vi "Boolean Debounce.vi"(1 "Reset":bool, 2 "Miliseconds":dbl, 3 "In":bool) -> (0 "Debounced":bool)   [LabVIEW 2016]
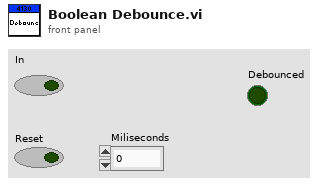
[diagram p1: front panel]
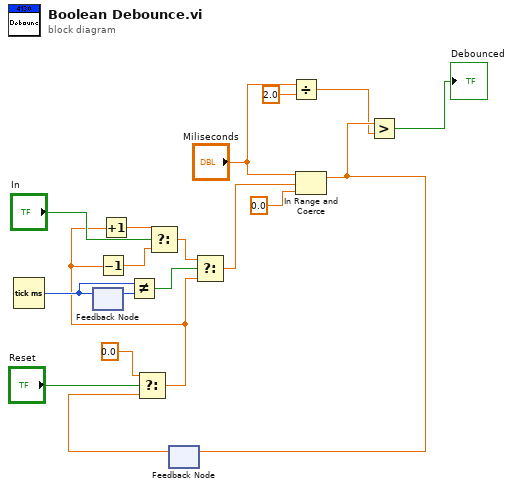
[diagram p0: block diagram]
diagram:
  n1 = Tick Count (ms)() -> (millisecond timer value=w4:u32)
  n2 = feedback-in #1(w4) -> ()
  n3 = feedback #1() -> (w5:u32)  [unwired: 1 in]
  n4 = Not Equal?(x=w4, y=w5) -> (x != y?=w3:bool)
  n5 = feedback #2() -> (w9:dbl)  [unwired: 1 in]
  n6 = Select(t=0.0, s="Reset", f=w9) -> (s? t:f=w1:dbl)
  n7 = Decrement(x=w1) -> (x-1=w17:dbl)
  n8 = Increment(x=w1) -> (x+1=w16:dbl)
  n9 = Select(t=w16, s="In", f=w17) -> (s? t:f=w2:dbl)
  n10 = Select(t=w2, s=w3, f=w1) -> (s? t:f=w6:dbl)
  n11 = Divide(x="Miliseconds", y=2.0) -> (x/y=w13:dbl)
  n12 = In Range and Coerce(upper limit="Miliseconds", x=w6, lower limit=0.0) -> (coerced(x)=w14:dbl)  [unwired: 1 out]
  n13 = feedback-in #2(w14) -> ()
  n14 = Greater?(x=w14, y=w13) -> (0:→"Debounced":bool)
